vi "EV Read Serial Atmosphere.vi"(0 "Run Step Inputs":T1={"Data in"=[], "Results in"=[], "Seq Setup in"="", "Step name"="", "Hardware in"="", "Calibration in"="", "Step # in sequence"=0, "Display step?(f)"=TRUE, "Generate names only"=FALSE, "Waveforms in"=[], "Memory List Grouping info"=[]} {"Waveforms in"."Y dB ref" format="%.1f"; "Waveforms in"."Y axis" items=["dB", "Lin", "Pwr"]; "Waveforms in"."Y data" items=["dB", "Lin", "Pwr"]; "Waveforms in"."X data" items=["dB", "Lin", "Pwr"]; "Data in"."Z data" items=["dB", "Lin", "Pwr"]; "Data in"."X data" items=["dB", "Lin", "Pwr"]; "Data in"."Y data" items=["dB", "Lin", "Pwr"]; "Data in"."Z dB ref" format="%.1f"; "Data in"."Z axis" items=["Log", "Lin"]; "Data in"."X dB ref" format="%.1f"; "Data in"."X axis" items=["Log", "Lin"]; "Data in"."Y axis" items=["Log", "Lin"]; "Data in"."Y dB ref" format="%.1f"; "Data in"."Curve"."z" format="%.2f"; "Data in"."Curve"."y" format="%.2f"; "Data in"."Curve"."x" format="%.2f"; "Results in"."Unit type" items=["dB", "Lin", "Pwr"]; "Results in"."Margin" format="%.2f"}, 11 "error in (no error)":errorcluster) -> (6 "Data out":T2 {"Z data" items=["dB", "Lin", "Pwr"]; "X data" items=["dB", "Lin", "Pwr"]; "Y data" items=["dB", "Lin", "Pwr"]; "Z dB ref" format="%.1f"; "Z axis" items=["Log", "Lin"]; "X dB ref" format="%.1f"; "X axis" items=["Log", "Lin"]; "Y axis" items=["Log", "Lin"]; "Y dB ref" format="%.1f"; "Curve"."z" format="%.2f"; "Curve"."y" format="%.2f"; "Curve"."x" format="%.2f"}, 8 "Results out":T5 {"Unit type" items=["dB", "Lin", "Pwr"]; "Margin" format="%.2f"}, 10 "Waveforms out":T7 {"Y dB ref" format="%.1f"; "Y axis" items=["dB", "Lin", "Pwr"]; "Y data" items=["dB", "Lin", "Pwr"]; "X data" items=["dB", "Lin", "Pwr"]}, 15 "error out":errorcluster)   [LabVIEW 2014]
uses:
  custom and SC Run Seq Sub VIs (x64).llb/data array.ctl
  custom and SC Run Seq Sub VIs (x64).llb/data cluster.ctl
  custom and SC Run Seq Sub VIs (x64).llb/Axis Unit Type.ctl
  custom and SC Run Seq Sub VIs (x64).llb/result array.ctl
  custom and SC Run Seq Sub VIs (x64).llb/result cluster.ctl
  custom and SC Run Seq Sub VIs (x64).llb/waveform array.ctl
  custom and SC Run Seq Sub VIs (x64).llb/waveform cluster.ctl
  custom and SC Run Seq Sub VIs (x64).llb/Run Step Inputs.ctl
  custom and SC Run Seq Sub VIs (x64).llb/Memory List Grouping.ctl
  custom and SC Run Seq Sub VIs (x64).llb/Memory List Grouping - Item Type.ctl
  custom and SC Run Seq Sub VIs (x64).llb/window stack manager Functions.ctl
  C:/SoundCheck 15.0-x64/System/Custom VIs/EV.Rotator.RotatorControl.dll
  EV.Rotator.RotatorControl.dll
panel:
  out "Humidity_Pct":dbl
  out "Pressure_kPa":dbl
  out "Temp_C":dbl
  # "NOTE:  These controls and indicators must stay here, but you can Hide them if you wish.  These are wired as the standard input/output connector pane for step run VIs."
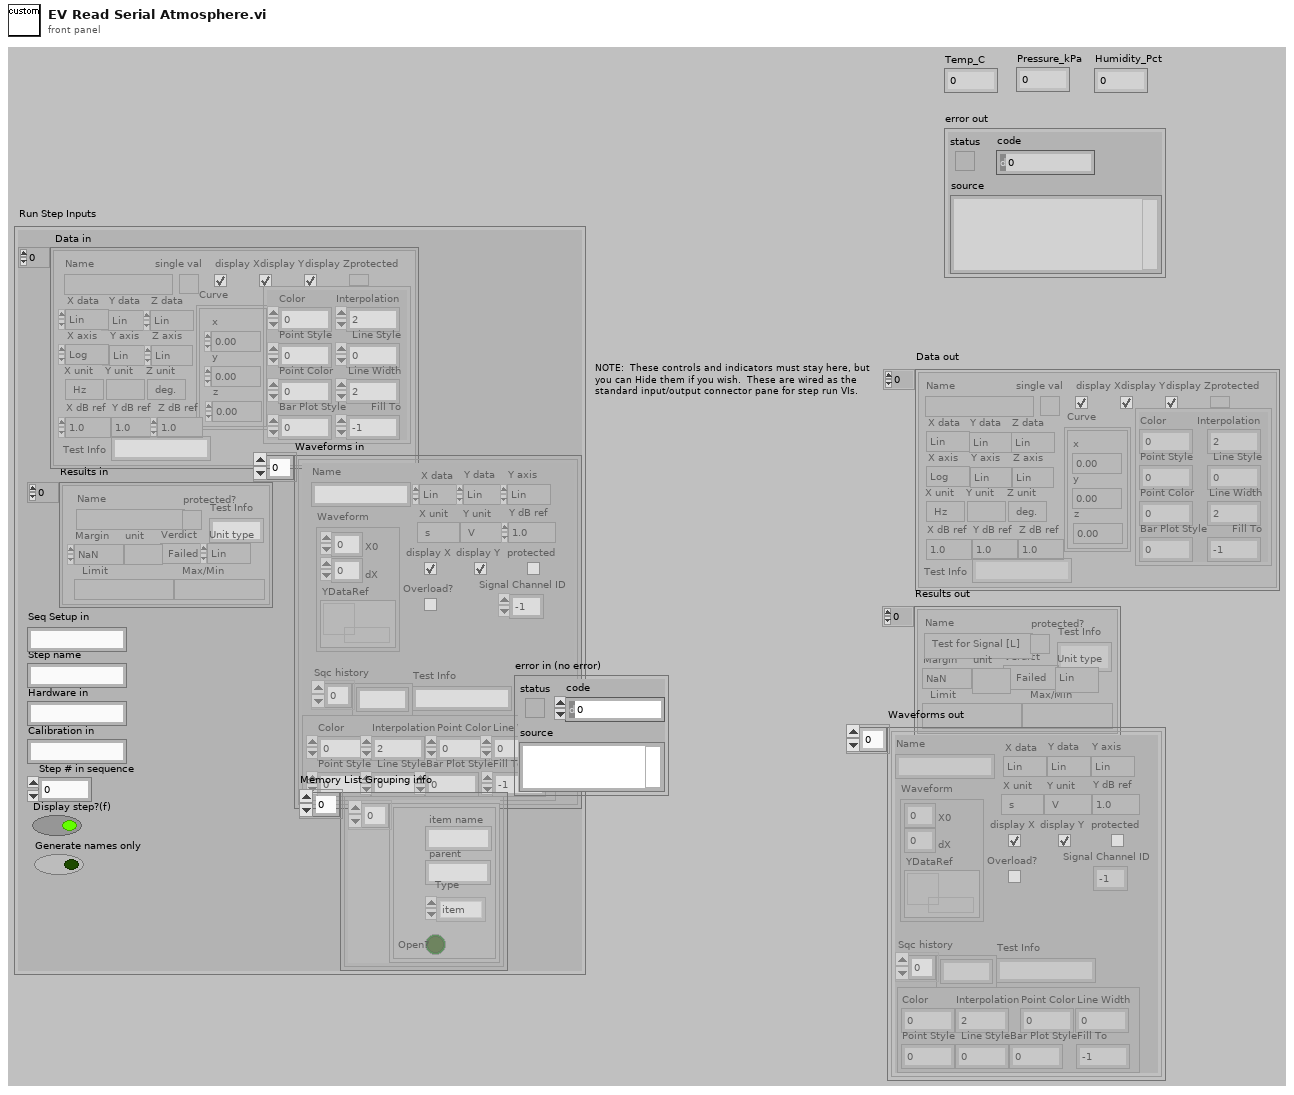
[diagram p1: front panel]
types:
  T1 = typedef "Run Step Inputs.ctl" = cluster{"Data in":T2, "Results in":T5, "Seq Setup in":string, "Step name":string, "Hardware in":string, "Calibration in":string, "Step # in sequence":i32, "Display step?(f)":bool, "Generate names only":bool, "Waveforms in":T7, "Memory List Grouping info":cluster{T9[]}[]}
  T2 = typedef "data array.ctl" = T3[]
  T3 = typedef "data cluster.ctl" = cluster{"Name":string, "Curve":cluster{"x":dbl, "y":dbl, "z":dbl}[], "X data":T4, "Y data":T4, "Z data":T4, "X axis":u16, "Y axis":u16, "Z axis":u16, "X unit":string, "Y unit":string, "Z unit":string, "X dB ref":dbl, "Y dB ref":dbl, "Z dB ref":dbl, "single val":bool, "protected":bool, "display X":bool, "display Y":bool, "display Z":bool, "Plot Settings":cluster{"Color":u32, "Interpolation":u8, "Point Style":u8, "Line Style":u8, "Point Color":u32, "Line Width":u8, "Bar Plot Style":u8, "Fill To":i16}, "Test Info":string}
  T4 = typedef "Axis Unit Type.ctl" = u16
  T5 = typedef "result array.ctl" = T6[]
  T6 = typedef "result cluster.ctl" = cluster{"Name":string, "Margin":dbl, "unit":string, "Verdict":bool, "Limit":string, "Max/Min":string, "protected?":bool, "Test Info":string, "Unit type":T4}
  T7 = typedef "waveform array.ctl" = T8[]
  T8 = typedef "waveform cluster.ctl" = cluster{"Name":string, "Waveform":cluster{"X0":dbl, "dX":dbl, "YDataRef":refnum<data-value>}, "X data":T4, "Y data":T4, "Y axis":T4, "X unit":string, "Y unit":string, "Y dB ref":dbl, "display Y":bool, "display X":bool, "Overload?":bool, "protected":bool, "Sqc history":string[], "Signal Channel ID":i32, "Plot Settings":cluster{"Color":u32, "Interpolation":u8, "Point Style":u8, "Line Style":u8, "Point Color":u32, "Line Width":u8, "Bar Plot Style":u8, "Fill To":i16}, "Test Info":string}
  T9 = typedef "Memory List Grouping.ctl" = cluster{"item name":string, "parent":string, "Open?":bool, "Type":T10}
  T10 = typedef "Memory List Grouping - Item Type.ctl" = enum16{"item", "custom group", "auto group", "protected group"}
  T11 = typedef "window stack manager Functions.ctl" = enum16{"Init", "add", "remove", "run", "clear", "vi stopped offset", "minimize all", "restore all", "autoadd", "Hourglass On", "Hourglass Off"}
  T12 = typedef "seq step setup.ctl" = cluster{"Input Signal Channels":i32[], "Output Signal Channels":i32[], "Curves selected":string[][], "Curves generated":string[], "Step setup flat":string, "Trigger Signal Channel":i32, "Curves Generated Assumptions":cluster{"seq-setup in":string, "Relevant subset of mem list Grouping":cluster{T9[]}[]}}
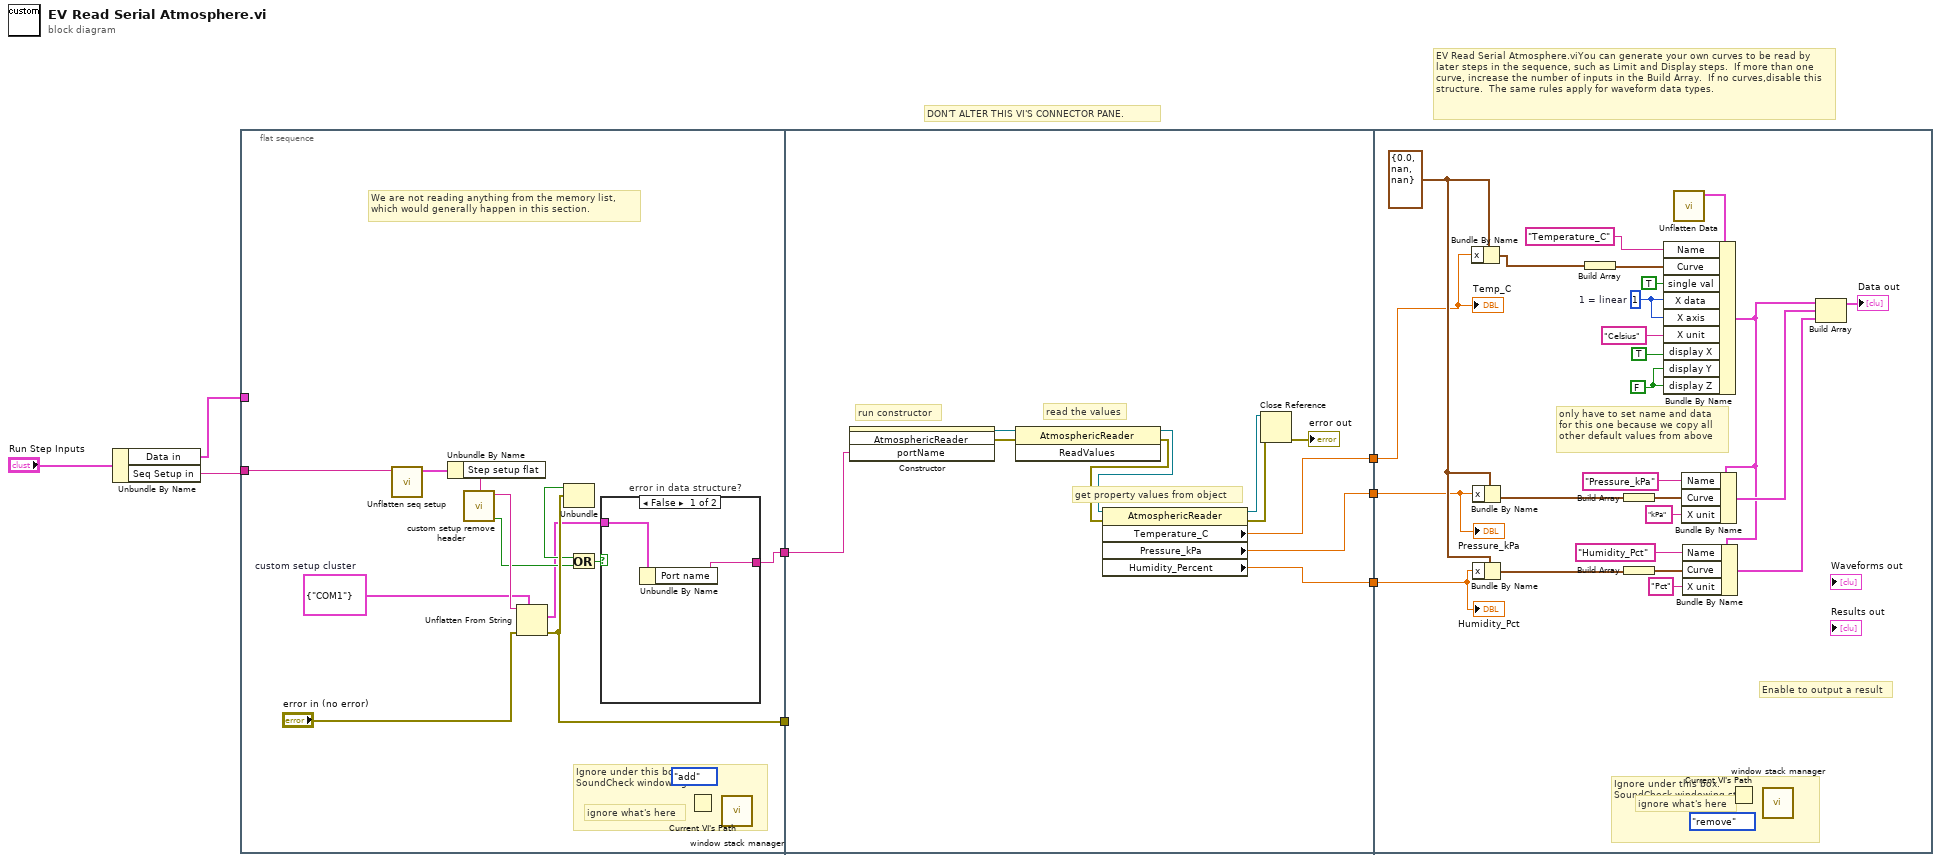
[diagram p0: block diagram]
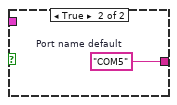
[diagram p2: hidden frame]
diagram:
  # "EV Read Serial Atmosphere.viYou can generate your own curves to be read by later steps in the sequence, such as Limit and Display steps.  If more than one curve, increase the number of inputs in the Build Array.  If no curves,disable this structure.  The same rules apply for waveform data types."
  # "DON'T ALTER THIS VI'S CONNECTOR PANE."
  n1 = Unbundle By Name("Run Step Inputs") -> ("Data in"=w3:T2, "Seq Setup in"=w2:string)
  n2 = flat-sequence {
    tunnel: w3 -> [_]
    tunnel: w2 -> [w21]
    tunnel: [w19] -> w7
    tunnel: [w20] -> w6
    tunnel: w7 -> [_]
    tunnel: w6 -> [w26]
    tunnel: [w31] -> w5
    tunnel: [w32] -> w4
    tunnel: [w33] -> w1
    tunnel: w5 -> [w37]
    tunnel: w4 -> [w39]
    tunnel: w1 -> [w38]
    frame #0 {
      w9 = cluster{"Port name":string} {"Port name"="COM1"}  # custom setup cluster
      # "We are not reading anything from the memory list,\nwhich would generally happen in this section."
      # "Ignore under this box. \nSoundCheck windowing stuff."
      # "ignore what's here"
      n3 = call "Unflatten seq setup.vi"("Unflatten seq setup"=w21) -> ("Sequence-specific step set-up"=w17:T12)  [unwired: 3 in, 7 out]
      n4 = Unbundle By Name(w17) -> ("Step setup flat"=w16:string)
      n5 = call "custom setup remove header.vi"("Output from 'Step setup flat' of seq-setup structure"=w16) -> ("Error?"=w14:bool, "Flattened custom step setup cluster"=w15:string)  [unwired: 9 out]
      n6 = Unflatten From String(type=w9, binary string=w15, error in (no error)="error in (no error)") -> (value=w11:cluster{"Port name":string}, error out=w19:errorcluster)  [unwired: 3 out]
      n7 = Unbundle(w19) -> ("status"=w13:bool)  [unwired: 2 out]
      n8 = Or(x=w13, y=w14) -> (x .or. y?=w12:bool)
      n9 = case "error in data structure?" shown="False" w12 {
        tunnel: [w24 w25] -> w20
        tunnel: w11 -> [w23 _]
        frame False {
          n10 = Unbundle By Name(w23) -> ("Port name"=w24:string)
        }
        frame True {
          w25 = "COM5"  # Port name default
        }
      }
      n11 = Current VI's Path() -> (path=w22:path)
      n12 = call "window stack manager.vi"("VI path"=w22, "Function (run)"=window_stack_manager_Functions."add") -> ()  [unwired: 5 in, 5 out]
    }
    frame #1 {
      # "get property values from object"
      # "read the values"
      # "run constructor"
      n13 = constructor class="AtmosphericReader"("portName"=w26) -> (reference out=w27:refnum<k24>, error out=w28:errorcluster)  [unwired: 3 in, 2 out]
      n14 = invoke class="AtmosphericReader" method="ReadValues"(reference=w27, error in=w28) -> (reference out=w30:refnum<k24>, error out=w29:errorcluster)  [unwired: 1 in, 1 out]
      n15 = property class="AtmosphericReader"(reference=w30, error in=w29) -> (reference out=w35:refnum<k24>, error out=w34:errorcluster, "Temperature_C"=w31:dbl, "Pressure_kPa"=w32:dbl, "Humidity_Percent"=w33:dbl)
      n16 = Close Reference(reference=w35, error in (no error)=w34) -> (error out=→"error out":errorcluster)
    }
    frame #2 {
      w55 = FALSE ("display Y")
      w47 = cluster{"x":dbl, "y":dbl, "z":dbl} {"x"=0.0, "y"=nan, "z"=nan}
      w54 = u16 1  # 1 = linear
      # "Ignore under this box. \nSoundCheck windowing stuff."
      # "only have to set name and data\nfor this one because we copy all\nother default values from above"
      # "ignore what's here"
      # "Enable to output a result"
      n17 = Bundle By Name(cluster=w47, "x"=w37) -> (w60:cluster{"x":dbl, "y":dbl, "z":dbl})
      n18 = Bundle By Name(cluster=w47, "x"=w39) -> (w53:cluster{"x":dbl, "y":dbl, "z":dbl})
      n19 = Bundle By Name(cluster=w47, "x"=w38) -> (w46:cluster{"x":dbl, "y":dbl, "z":dbl})
      n20 = Build Array(w60) -> (w59:cluster{"x":dbl, "y":dbl, "z":dbl}[])
      n21 = Build Array(w53) -> (w52:cluster{"x":dbl, "y":dbl, "z":dbl}[])
      n22 = Build Array(w46) -> (w42:cluster{"x":dbl, "y":dbl, "z":dbl}[])
      n23 = call "Unflatten Data.vi"() -> ("Datum"=w61:T3)  [unwired: 1 in, 10 out]
      n24 = Bundle By Name(cluster=w61, "Name"="Temperature_C" ("Bundle Element"), "Curve"=w59, "single val"=TRUE ("T = data is just a single number (the Y element)"), "X data"=w54, "X axis"=w54, "X unit"="Celsius", "display X"=TRUE, "display Y"=w55, "display Z"=w55) -> (w40:T3)
      n25 = Bundle By Name(cluster=w40, "Name"="Pressure_kPa" ("Bundle Element"), "Curve"=w52, "X unit"="kPa") -> (w51:T3)
      n26 = Bundle By Name(cluster=w40, "Name"="Humidity_Pct" ("Bundle Element"), "Curve"=w42, "X unit"="Pct") -> (w41:T3)
      n27 = Current VI's Path() -> (path=w62:path)
      n28 = call "window stack manager.vi"("VI path"=w62, "Function (run)"=window_stack_manager_Functions."remove") -> ()  [unwired: 5 in, 5 out]
      n29 = Build Array(w40, w51, w41) -> (→"Data out":T3[])
      "Temp_C" <- w37
      "Pressure_kPa" <- w39
      "Humidity_Pct" <- w38
    }
  }
